vi "波形图表.vi"() -> ()   [LabVIEW 2018]
panel:
  out "波形图表 2":T1(graph)
  in  "停止":bool
  out "波形图表":dbl[][](graph)
  out "波形图":dbl[][](graph)
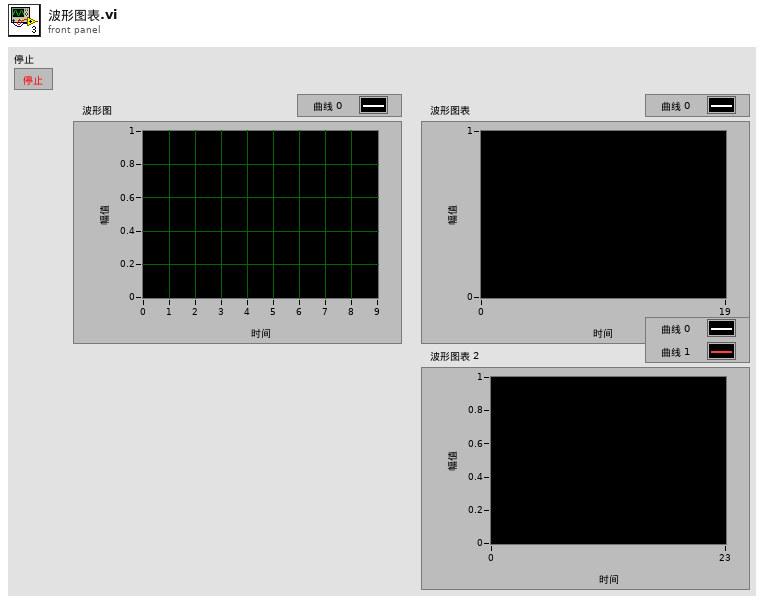
[diagram p1: front panel]
types:
  T1 = cluster{"number: 0 to 1":dbl, "number: 0 to 1":dbl}
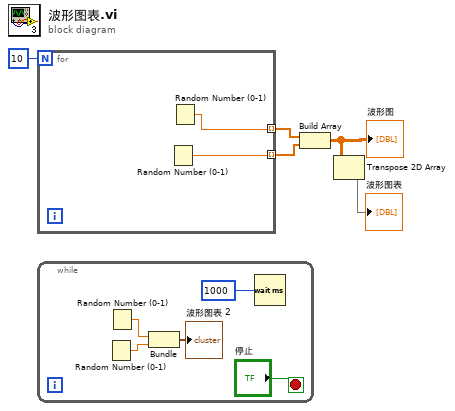
[diagram p0: block diagram]
diagram:
  n1 = for {
    N: 10 -> [_]
    tunnel: [w7] -> w4 mode=indexing
    tunnel: [w6] -> w3 mode=indexing
    n2 = Random Number (0-1)() -> (number: 0 to 1=w6:dbl)
    n3 = Random Number (0-1)() -> (number: 0 to 1=w7:dbl)
  }
  n4 = while {
    stop <- "停止" stop-if-true
    n5 = Random Number (0-1)() -> (number: 0 to 1=w10:dbl)
    n6 = Random Number (0-1)() -> (number: 0 to 1=w11:dbl)
    n7 = Bundle("number: 0 to 1"=w11, "number: 0 to 1"=w10) -> (→"波形图表 2":T1)  [unwired: 1 in]
    n8 = Wait (ms)(milliseconds to wait=u32 1000 ("毫秒计时值")) -> ()  [unwired: 1 out]
  }
  n9 = Build Array(w4, w3) -> (w2:dbl[][])
  "波形图" <- w2
  n10 = Transpose 2D Array(2D array=w2) -> (transposed array=→"波形图表":dbl[][])
